vi "read_data_from_tdms_file.vi"(0 "chemin du fichier":path) -> (1 "capteur1":waveform(dbl), 2 "capteur2":waveform(dbl), 3 "capteur3":waveform(dbl), 4 "capteur4":waveform(dbl))   [LabVIEW 2020]
panel:
  out "données":waveform(dbl)[](array[waveform])
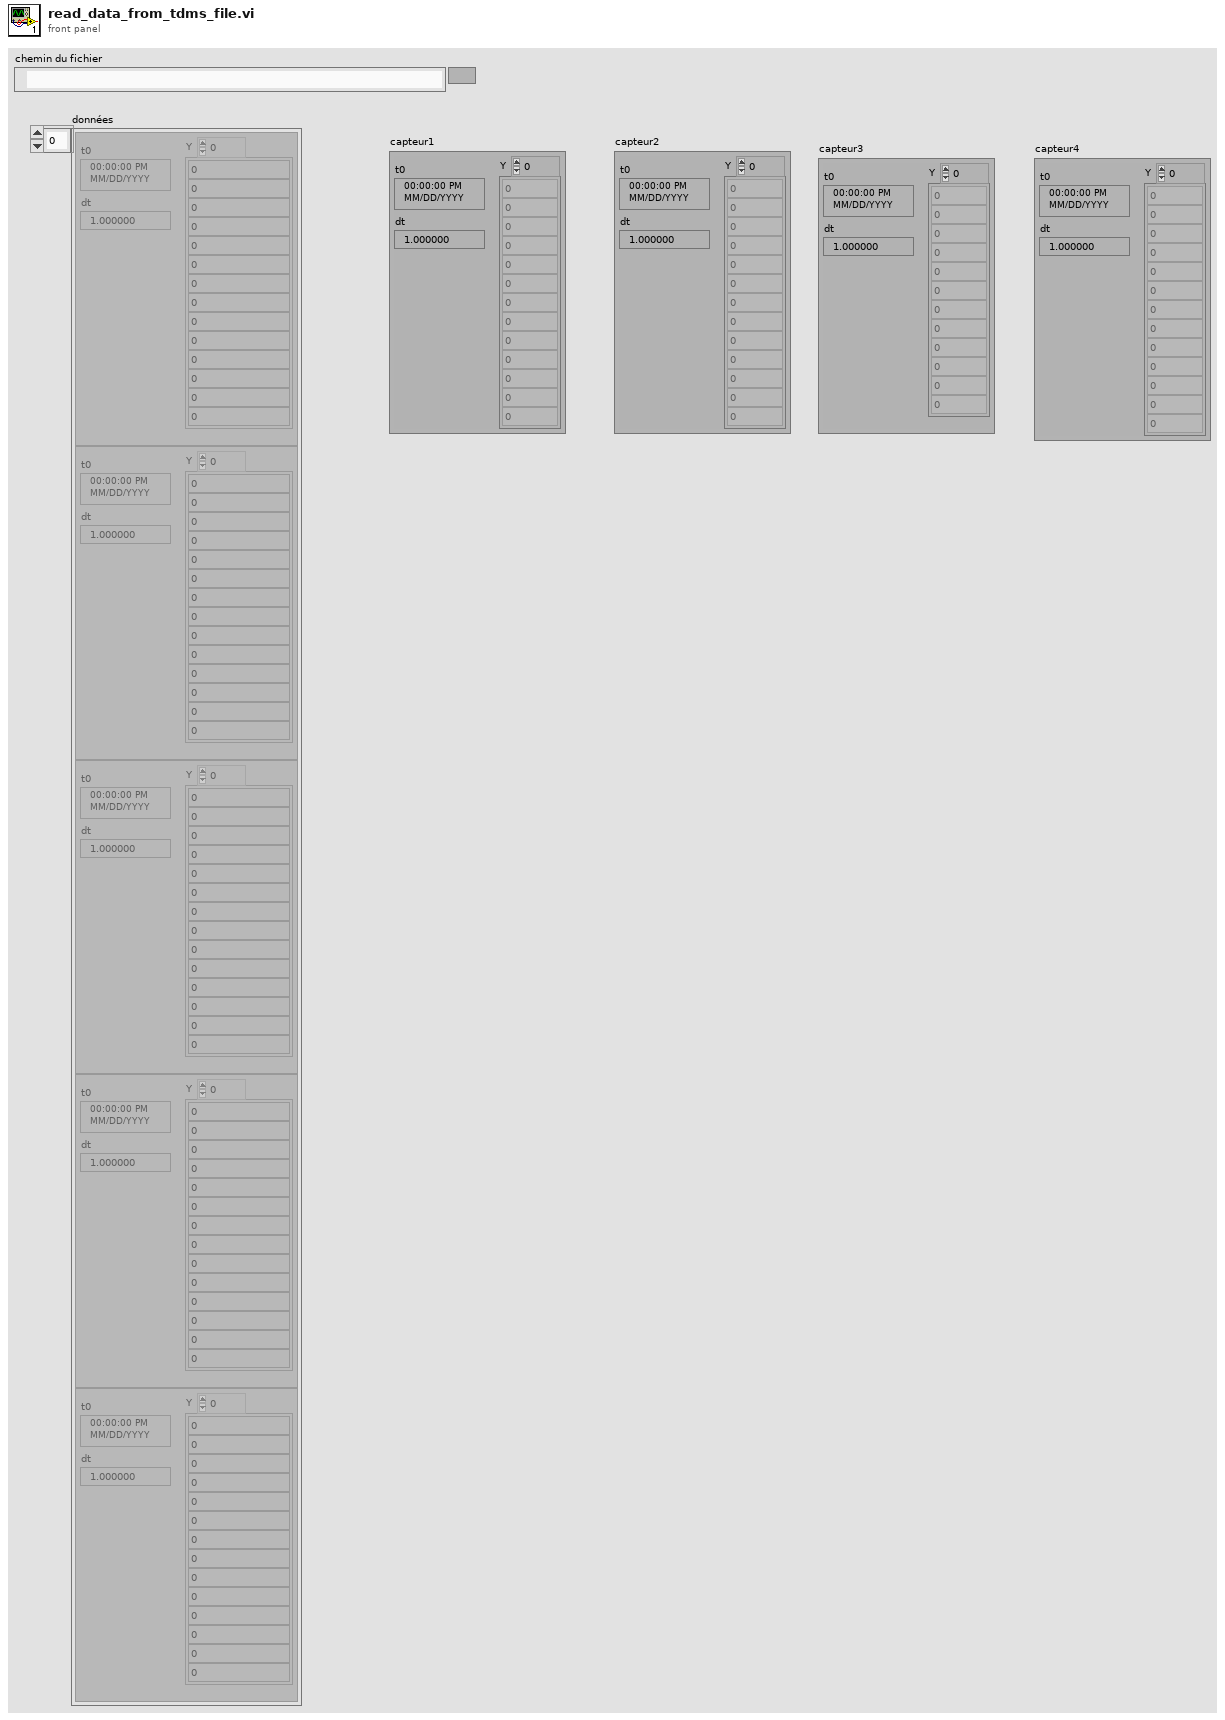
[diagram p1: front panel]
types:
  T1 = cluster{"data[0]":waveform(dbl), "data[1]":waveform(dbl), "data[2]":waveform(dbl), "data[3]":waveform(dbl), "data[4]":waveform(dbl), "data[5]":waveform(dbl), "data[6]":waveform(dbl), "data[7]":waveform(dbl), "data[8]":waveform(dbl)}
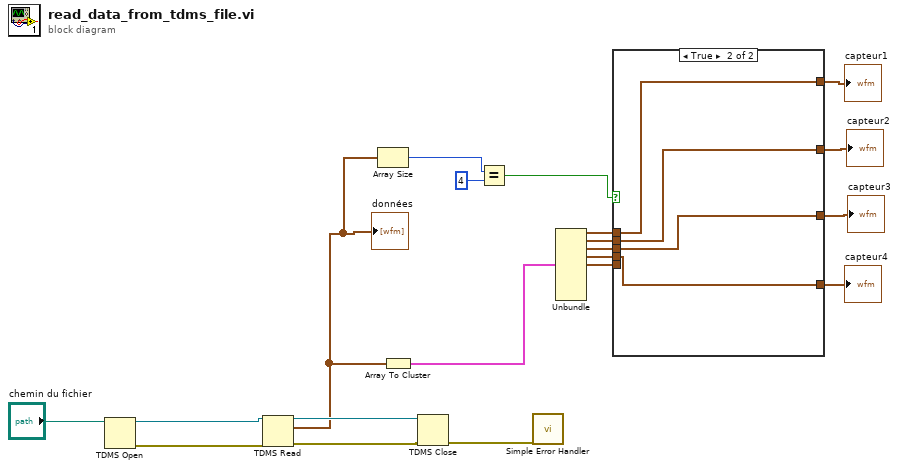
[diagram p0: block diagram]
diagram:
  n1 = TDMS Open(11:"chemin du fichier") -> (0:w20:errorcluster, 3:w16:refnum<k34>)  [unwired: 6 in]
  n2 = TDMS Read(0:w16, 11:w20) -> (4:w15:refnum<k34>, 10:w13:waveform(dbl)[], 15:w19:errorcluster)  [unwired: 6 in, 3 out]
  "données" <- w13
  n3 = Array Size(array=w13) -> (size(s)=w12:i32)
  n4 = Array To Cluster(array=w13) -> (cluster=w14:T1)
  n5 = TDMS Close(8:w19, 11:w15) -> (0:w18:errorcluster)  [unwired: 1 out]
  n6 = Equal?(x=w12, y=4) -> (x = y?=w10:bool)
  n7 = call <vilib>:"Simple Error Handler.vi"("error in (no error)"=w18) -> ()  [unwired: 4 in, 5 out]
  n8 = Unbundle(w14) -> ("data[0]"=w8:waveform(dbl), "data[1]"=w7:waveform(dbl), "data[2]"=w5:waveform(dbl), "data[3]"=w2:waveform(dbl), "data[4]"=w1:waveform(dbl))  [unwired: 4 out]
  n9 = case shown="True" w10 {
    tunnel: [w24 w28] -> w9
    tunnel: w8 -> [_ w28]
    tunnel: w7 -> [w24 w27]
    tunnel: [w23 w27] -> w6
    tunnel: w5 -> [w23 w26]
    tunnel: [w22 w26] -> w4
    tunnel: [w21 w25] -> w3
    tunnel: w2 -> [w22 w25]
    tunnel: w1 -> [w21 _]
    frame False {
    }
    frame True {
    }
  }
  "capteur1" <- w9
  "capteur2" <- w6
  "capteur4" <- w3
  "capteur3" <- w4
